vi "Roughness Averager Peak Density Compute.vi"(8 "error in (no error)":errorcluster, 10 "Grayscale Image":T1, 11 "Roughness Averager in":refnum<class "Roughness Averager.lvclass">) -> (0 "error out":errorcluster, 3 "Roughness Averager out":refnum<class "Roughness Averager.lvclass">)   [LabVIEW 2018, in "Roughness Averager.lvclass"]
uses:
  Roughness Averager.lvclass
  <vilib>/vision/Image Controls.llb/IMAQ Image.ctl
  Roughness Averager.lvclass/Roughness Averager.ctl
  a31f3be0-eb34-42fd-98b5-976c538d4073.vi
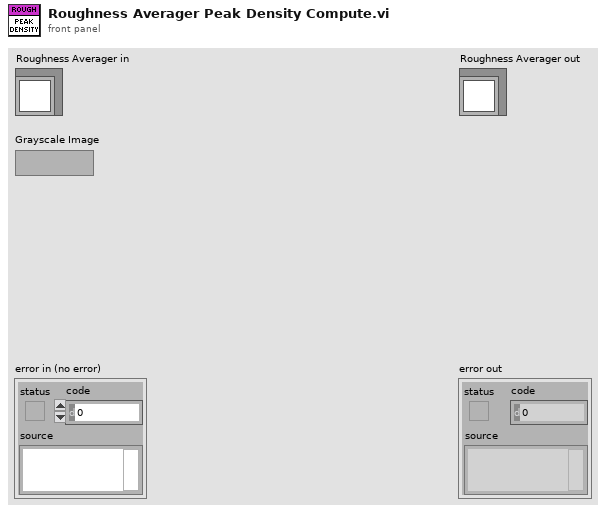
[diagram p1: front panel]
types:
  T1 = typedef "IMAQ Image.ctl" = refnum<image>
  T2 = typedef "Video Cam Processor.lvclass/Hull Point STYP.ctl" = cluster{"X":i32, "Y":i32}
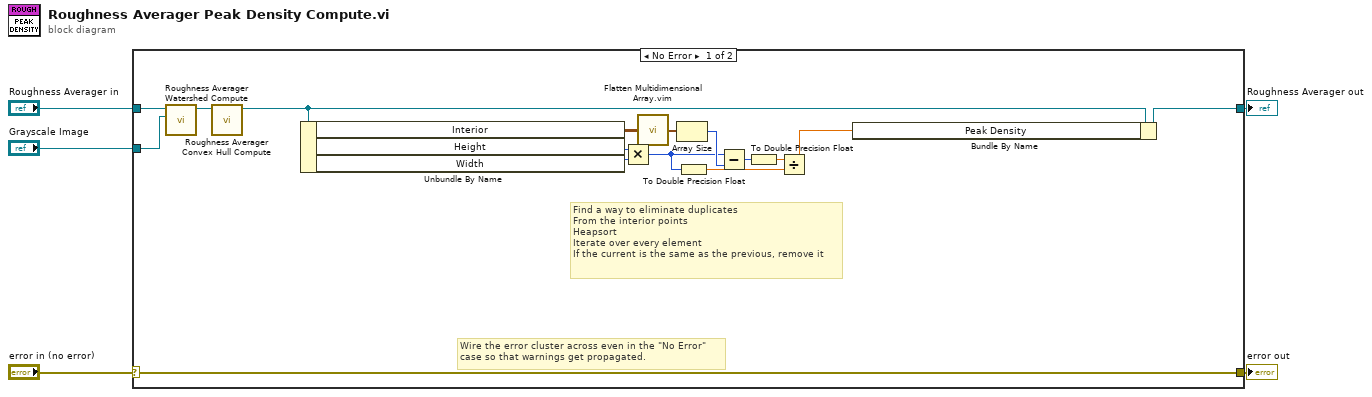
[diagram p0: block diagram]
diagram:
  n1 = case shown="No Error" "error in (no error)" {
    selector: "error in (no error)" -> [w21 w23]
    tunnel: [w21 w23] -> w4
    tunnel: [w10 w22] -> w2
    tunnel: "Roughness Averager in" -> [w9 w22]
    tunnel: "Grayscale Image" -> [w6 _]
    frame No Error {
      # "Find a way to eliminate duplicates\nFrom the interior points\nHeapsort\nIterate over every element\nIf the current is the same as the previous, remove it"
      # "Wire the error cluster across even in the \"No Error\"\ncase so that warnings get propagated."
      n2 = call-dynamic "Roughness Averager Watershed Compute.vi"("Grayscale Image"=w6, "Roughness Averager in"=w9) -> ("Roughness Averager out"=w8:refnum<class "Roughness Averager.lvclass">)  [unwired: 8 in, 1 out]
      n3 = call-dynamic "Roughness Averager Convex Hull Compute.vi"("Roughness Averager in"=w8) -> ("Roughness Averager out"=w7:refnum<class "Roughness Averager.lvclass">)  [unwired: 9 in, 1 out]
      n4 = Unbundle By Name(w7) -> ("Interior"=w20:T2[][], "Height"=w18:i32, "Width"=w17:i32)
      n5 = Multiply(x=w18, y=w17) -> (x*y=w13:i32)
      n6 = call "Flatten Multidimensional Array.vim"("Array"=w20) -> ("output array"=w19:T2[])  [unwired: 14 in]
      n7 = Array Size(array=w19) -> (size(s)=w16:i32)
      n8 = To Double Precision Float(number=w13) -> (double precision float=w12:dbl)
      n9 = Subtract(x=w13, y=w16) -> (x-y=w15:i32)
      n10 = To Double Precision Float(number=w15) -> (double precision float=w14:dbl)
      n11 = Divide(x=w14, y=w12) -> (x/y=w11:dbl)
      n12 = Bundle By Name(cluster=w7, "Peak Density"=w11) -> (w10:refnum<class "Roughness Averager.lvclass">)
    }
    frame Error {
    }
  }
  "error out" <- w4
  "Roughness Averager out" <- w2
